vi "Wavelet Transform Daubechies4 Inverse PtByPt.vi"(2 "initialize":bool, 3 "sample length":i32=128, 5 "x":dbl format="%0.2f") -> (0 "error":i32, 1 "Wavelet Daubechies4 Inv {X}":dbl[](array[numeric]))   [LabVIEW 2020, in "NI_PtbyPt.lvlib"]
doc: "Performs the inverse of the wavelet transform based on the Daubechies4 function."
uses:
  NI_PtbyPt.lvlib
  Real Dot Product.vi
  NI_AALBase.lvlib
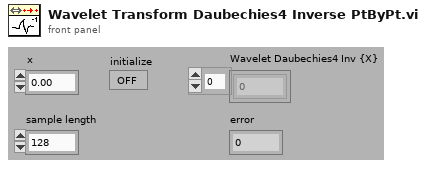
[diagram p1: front panel]
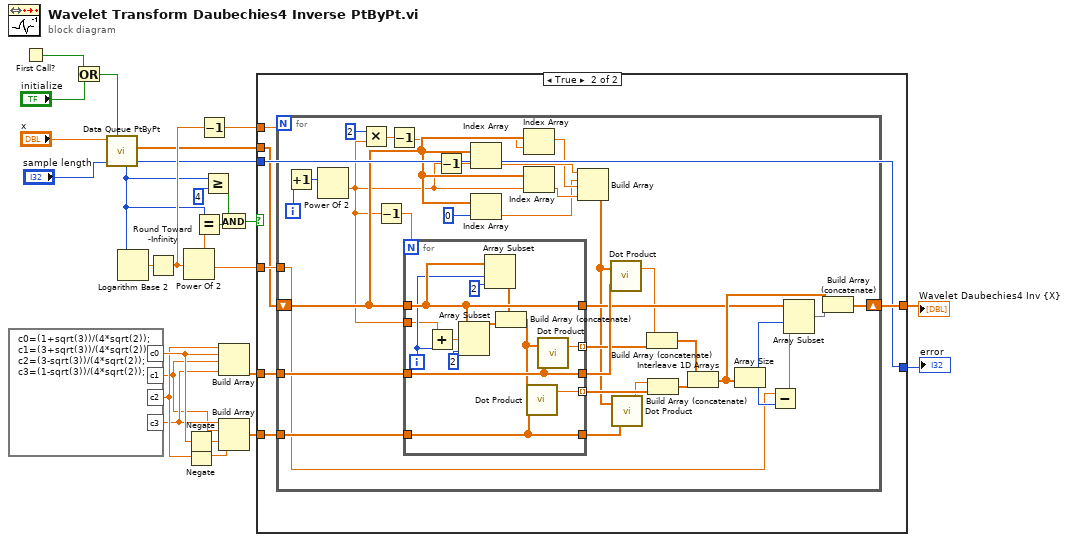
[diagram p0: block diagram]
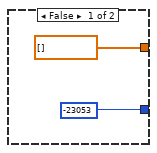
[diagram p2: hidden frame]
diagram:
  n1 = formula code="c0=(1+sqrt(3))/(4*sqrt(2));\nc1=(3+sqrt(3))/(4*sqrt(2));\nc2=(3-sqrt(3))/(4*sqrt(2));\nc3=(1-sqrt(3))/(4*sqrt(2));"() -> ("c0"=w17:dbl, "c1"=w14:dbl, "c2"=w16:dbl, "c3"=w15:dbl)
  n2 = First Call?() -> (First Call?: T/F=w4:bool)
  n3 = Or(x=w4, y="initialize") -> (x .or. y?=w3:bool)
  n4 = call "Data Queue PtByPt.vi"("initialize"=w3, "sample length"="sample length", "input data point"="x") -> ("error"=w2:i32, "Current Queue"=w1:dbl[], "current length"=w6:i32)  [unwired: 4 in, 2 out]
  n5 = Logarithm Base 2(1:w6) -> (0:w26:dbl)
  n6 = Round Toward -Infinity(1:w26) -> (0:w11:dbl)
  n7 = Power Of 2(x=w11) -> (2^x=w25:dbl)
  n8 = Negate(x=w17) -> (-x=w13:dbl)
  n9 = Negate(x=w16) -> (-x=w12:dbl)
  n10 = Equal?(x=w6, y=w25) -> (x = y?=w21:bool)
  n11 = Decrement(x=w11) -> (x-1=w10:dbl)
  n12 = Greater Or Equal?(x=w6, y=4) -> (x >= y?=w22:bool)
  n13 = And(x=w22, y=w21) -> (x .and. y?=w20:bool)
  n14 = Build Array(w16, w17, w14, w15) -> (w19:dbl[])
  n15 = Build Array(w15, w14, w13, w12) -> (w18:dbl[])
  n16 = case shown="True" w20 {
    tunnel: [-23053 w30] -> w24
    tunnel: w10 -> [_ w31]
    tunnel: w19 -> [_ w35]
    tunnel: w18 -> [_ w34]
    tunnel: w25 -> [_ w33]
    tunnel: [dbl[] [] ("Current Queue") w32] -> w9
    tunnel: w2 -> [_ w30]
    tunnel: w1 -> [_ w29]
    frame False {
    }
    frame True {
      n17 = for {
        N: w31 -> [_]
        shift-right: [w39] -> w32
        shift-left: w29 -> [w46]
        tunnel: w35 -> [w67]
        tunnel: w34 -> [w66]
        tunnel: w33 -> [w45]
        i -> [w37]
        n18 = Increment(x=w37) -> (x+1=w36:i32)
        n19 = Power Of 2(x=w36) -> (2^x=w38:dbl)
        n20 = Multiply(x=2, y=w38) -> (x*y=w42:dbl)
        n21 = Decrement(x=w38) -> (x-1=w47:dbl)
        n22 = Decrement(x=w42) -> (x-1=w40:dbl)
        n23 = for {
          N: w47 -> [_]
          tunnel: w46 -> [w76]
          tunnel: w67 -> [w79]
          tunnel: w66 -> [w78]
          tunnel: [w76] -> w60
          tunnel: [w79] -> w65
          tunnel: [w78] -> w64
          tunnel: [w72] -> w54 mode=indexing
          tunnel: [w71] -> w53 mode=indexing
          tunnel: w38 -> [w69]
          i -> [w70]
          n24 = Add(x=w69, y=w70) -> (x+y=w68:dbl)
          n25 = Array Subset(array=w76, index=w68, length=2) -> (w74:dbl[])
          n26 = Array Subset(array=w76, index=w70, length=2) -> (w75:dbl[])
          n27 = Build Array (concatenate)(w75, w74) -> (w73:dbl[])
          n28 = call-poly "Dot Product.vi"("Y Vector"=w78, "X Vector"=w73) -> ("X * Y"=w71:dbl)  [unwired: 1 out]
          n29 = call-poly "Dot Product.vi"("Y Vector"=w79, "X Vector"=w73) -> ("X * Y"=w72:dbl)  [unwired: 1 out]
        }
        n30 = Decrement(x=w38) -> (x-1=w43:dbl)
        n31 = Index Array(array=w46, index=w43) -> (element=w58:dbl)
        n32 = Index Array(array=w46, index=0) -> (element=w49:dbl)
        n33 = Index Array(array=w46, index=w40) -> (element=w57:dbl)
        n34 = Index Array(array=w46, index=w38) -> (element=w56:dbl)
        n35 = Build Array(w58, w49, w57, w56) -> (w48:dbl[])
        n36 = call-poly "Dot Product.vi"("Y Vector"=w65, "X Vector"=w48) -> ("X * Y"=w55:dbl)  [unwired: 1 out]
        n37 = call-poly "Dot Product.vi"("Y Vector"=w64, "X Vector"=w48) -> ("X * Y"=w52:dbl)  [unwired: 1 out]
        n38 = Build Array (concatenate)(w55, w54) -> (w51:dbl[])
        n39 = Build Array (concatenate)(w52, w53) -> (w50:dbl[])
        n40 = Interleave 1D Arrays(w51, w50) -> (w62:dbl[])
        n41 = Array Size(array=w62) -> (size(s)=w61:i32)
        n42 = Subtract(x=w45, y=w61) -> (x-y=w44:dbl)
        n43 = Array Subset(array=w60, index=w61, length=w44) -> (w63:dbl[])
        n44 = Build Array (concatenate)(w62, w63) -> (w39:dbl[])
      }
    }
  }
  "error" <- w24
  "Wavelet Daubechies4 Inv {X}" <- w9
